vi "Benchmark SV Send  LV2012 - NI Verified - 1.vi"() -> ()   [LabVIEW 2015]
panel:
  out "number (0 to 1)":dbl
  in  "Reset":bool
  out "Tries":u32
  out "Average Delay (ms)":dbl
  out "Delay (ms)":u32
  in  "stop":bool
  in  "Time between sends (ms)":u32=100
  # "Overview:  Coding that exemplifies how to benchmark the communication of Shared Variables.\nRequirements: LabVIEW 2012 or compatible\nInstructions:\n1.  Run the \"Benchmark SV Receive LV2012 - NI Verified.vi\"\n2. Run this VI\n3. Watch the amount of time it takes to communicate\n4. Stop both VIs"
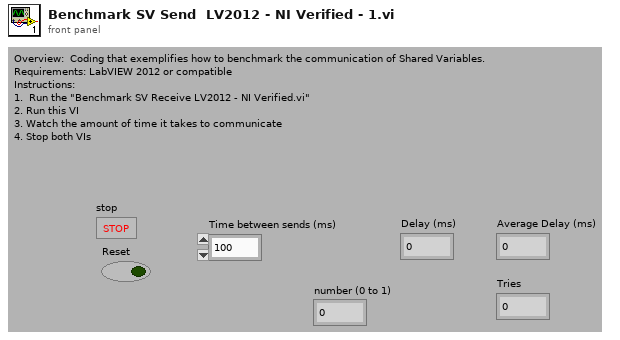
[diagram p1: front panel]
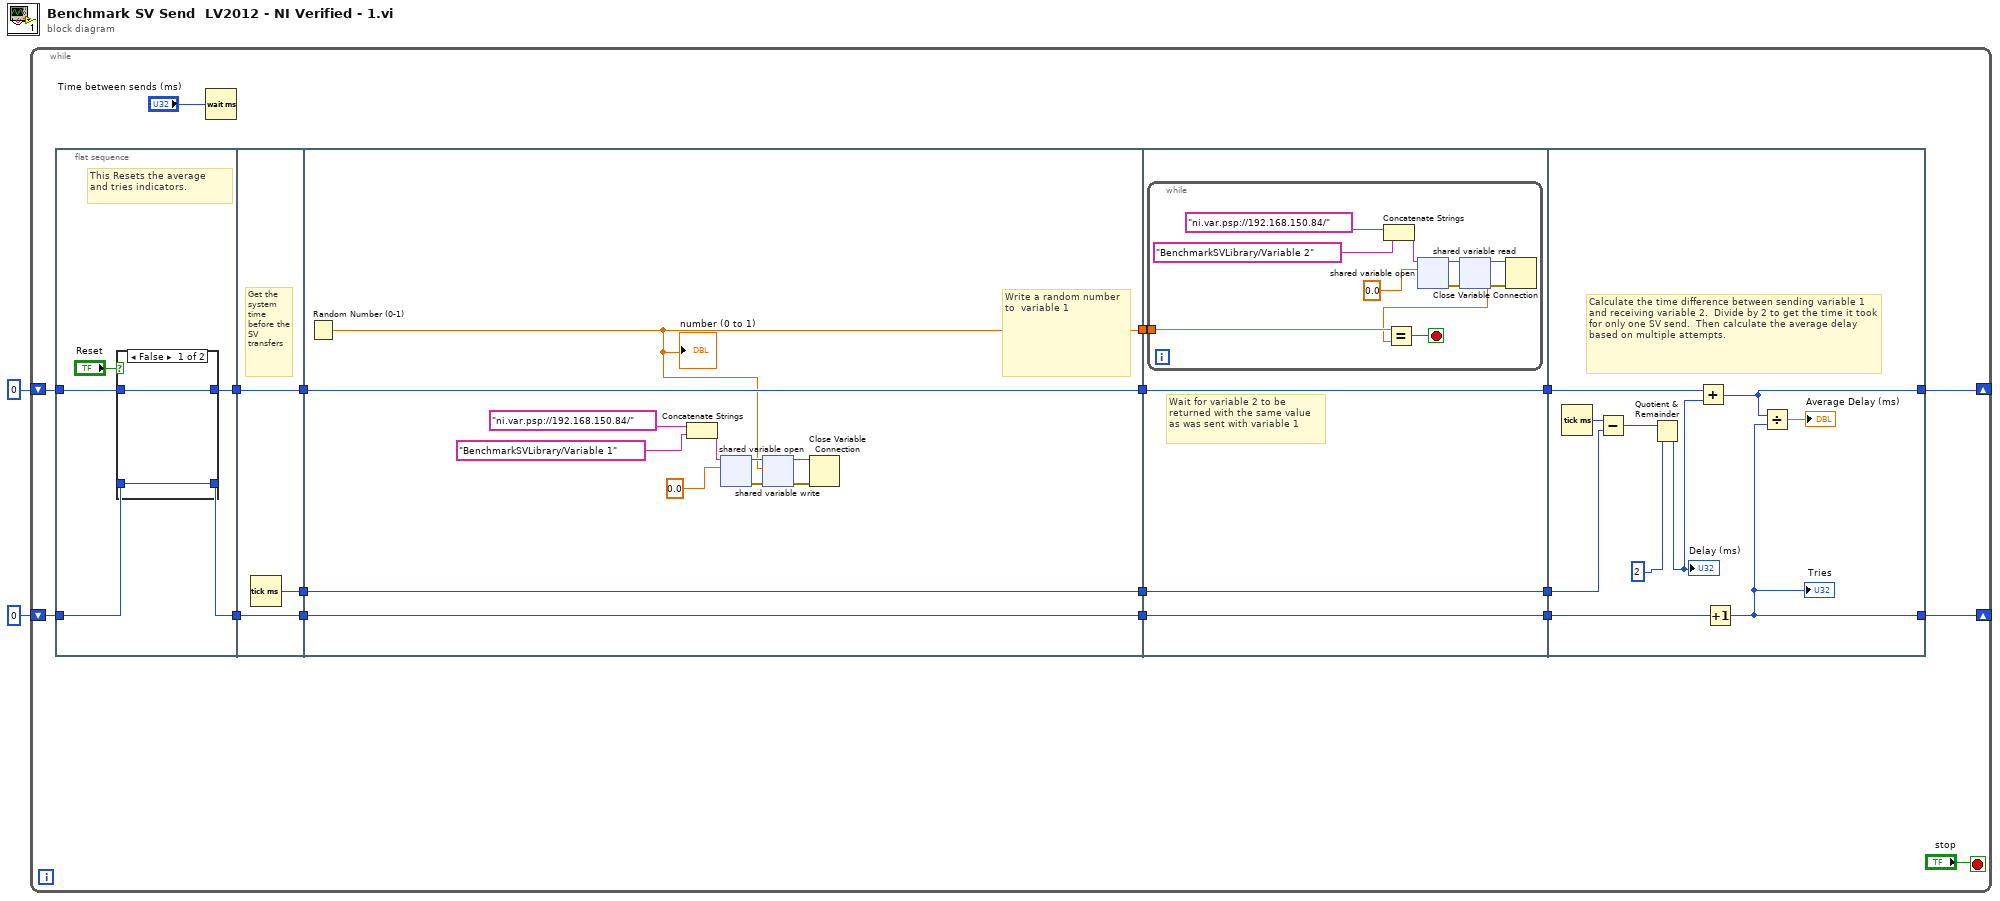
[diagram p0: block diagram]
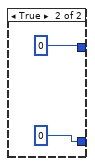
[diagram p2: hidden frame]
diagram:
  n1 = while {
    shift-right: [w15] -> _
    shift-left: u32 0 -> [w3]
    shift-right: [w12] -> _
    shift-left: u32 0 -> [w4]
    stop <- "stop" stop-if-true
    n2 = flat-sequence {
      tunnel: w3 -> [w25]
      tunnel: [w24] -> w8
      tunnel: [w22] -> w6
      tunnel: w4 -> [w21]
      tunnel: [w30] -> w9
      tunnel: w8 -> [w32]
      tunnel: [w32] -> w7
      tunnel: w6 -> [w31]
      tunnel: [w31] -> w5
      tunnel: [w33] -> w18
      tunnel: [w44] -> w17
      tunnel: [w43] -> w13
      tunnel: [w42] -> w10
      tunnel: w9 -> [w44]
      tunnel: w7 -> [w43]
      tunnel: w5 -> [w42]
      tunnel: w18 -> [w48]
      tunnel: [w47] -> w16
      tunnel: w17 -> [w47]
      tunnel: [w46] -> w14
      tunnel: w13 -> [w46]
      tunnel: [w45] -> w11
      tunnel: w10 -> [w45]
      tunnel: w16 -> [w68]
      tunnel: [w61] -> w15
      tunnel: w14 -> [w63]
      tunnel: [w60] -> w12
      tunnel: w11 -> [w67]
      frame #0 {
        # "This Resets the average \nand tries indicators."
        n3 = case shown="False" "Reset" {
          tunnel: [w27 u32 0] -> w24
          tunnel: w25 -> [w27 _]
          tunnel: [w26 u32 0] -> w22
          tunnel: w21 -> [w26 _]
          frame False {
          }
          frame True {
          }
        }
      }
      frame #1 {
        # "Get the system time before the SV transfers"
        n4 = Tick Count (ms)() -> (millisecond timer value=w30:u32)
      }
      frame #2 {
        # "Write a random number to  variable 1"
        n5 = Random Number (0-1)() -> (number: 0 to 1=w33:dbl)
        "number (0 to 1)" <- w33
        n6 = Concatenate Strings("ni.var.psp://192.168.150.84/" ("string"), "BenchmarkSVLibrary/Variable 1") -> (w36:string)
        n7 = shared-variable-open(w36, 0.0) -> (w40:refnum<k21>, w37:errorcluster)  [unwired: 2 in]
        n8 = shared-variable-write(w40, w37, w33) -> (w38:refnum<k21>, w39:errorcluster)
        n9 = Close Variable Connection(8:w39, 11:w38) -> ()  [unwired: 1 out]
      }
      frame #3 {
        # "Wait for variable 2 to be returned with the same value as was sent with variable 1"
        n10 = while {
          tunnel: w48 -> [w59]
          stop <- w58 stop-if-true
          n11 = Concatenate Strings("ni.var.psp://192.168.150.84/" ("string"), "BenchmarkSVLibrary/Variable 2") -> (w55:string)
          n12 = shared-variable-open(w55, 0.0) -> (w51:refnum<k21>, w54:errorcluster)  [unwired: 2 in]
          n13 = shared-variable-read(w51, w54) -> (w53:refnum<k21>, w52:errorcluster, w49:dbl)  [unwired: 1 out]
          n14 = Equal?(x=w59, y=w49) -> (x = y?=w58:bool)
          n15 = Close Variable Connection(8:w52, 11:w53) -> ()  [unwired: 1 out]
        }
      }
      frame #4 {
        # "Calculate the time difference between sending variable 1 and receiving variable 2.  Divide by 2 to get the time it took for only one SV send.  Then calculate the average delay based on multiple attempts."
        n16 = Tick Count (ms)() -> (millisecond timer value=w69:u32)
        n17 = Subtract(x=w69, y=w68) -> (x-y=w66:u32)
        n18 = Quotient & Remainder(x=w66, y=u32 2) -> (floor(x/y)=w64:u32)  [unwired: 1 out]
        "Delay (ms)" <- w64
        n19 = Add(x=w63, y=w64) -> (x+y=w61:u32)
        n20 = Increment(x=w67) -> (x+1=w60:u32)
        "Tries" <- w60
        n21 = Divide(x=w61, y=w60) -> (x/y=→"Average Delay (ms)":dbl)
      }
    }
    n22 = Wait (ms)(milliseconds to wait="Time between sends (ms)") -> ()  [unwired: 1 out]
  }
